vi "Feedback message.vi"(7 "Result":bool, 10 "error in (no error)":errorcluster, 11 "CMD Name":string) -> (2 "error out":errorcluster, 3 "Feedback":string)   [LabVIEW 2021, in "Model_AMC.lvclass"]
uses:
  Model_AMC.lvclass
  Model_AMC.lvclass/Model_AMC.ctl
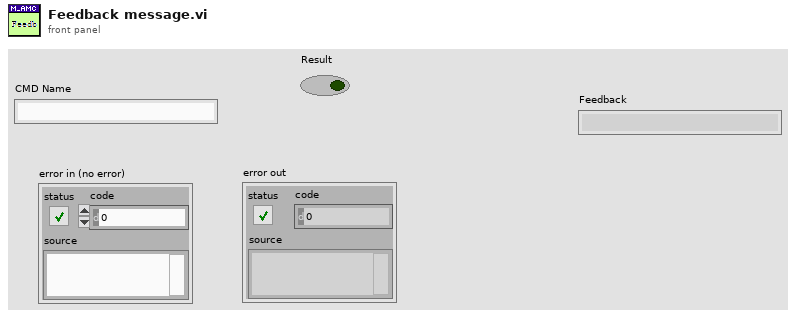
[diagram p1: front panel]
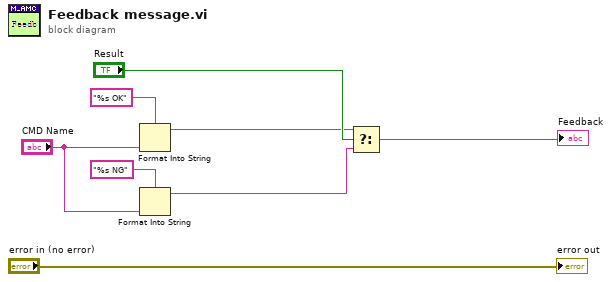
[diagram p0: block diagram]
diagram:
  n1 = Format Into String(format string="%s OK", "CMD Name") -> (resulting string=w5:string)  [unwired: 2 in, 1 out]
  n2 = Format Into String(format string="%s NG", "CMD Name") -> (resulting string=w2:string)  [unwired: 2 in, 1 out]
  n3 = Select(t=w5, s="Result", f=w2) -> (s? t:f=→"Feedback":string)
  "error out" <- "error in (no error)"
